vi "Run.vi"(8 "error in (no error)":errorcluster, 11 "Trigger in":refnum<class "Trigger.lvclass">) -> (0 "error out":errorcluster, 3 "Trigger out":refnum<class "Trigger.lvclass">)   [LabVIEW 2018, in "Trigger.lvclass"]
uses:
  Trigger.lvclass
  Trigger.lvclass/Trigger.ctl
  StateMachine/State Machine.lvclass
  Interface/Interface.lvclass
  Device/Device.lvclass
panel:
  out "resp":string
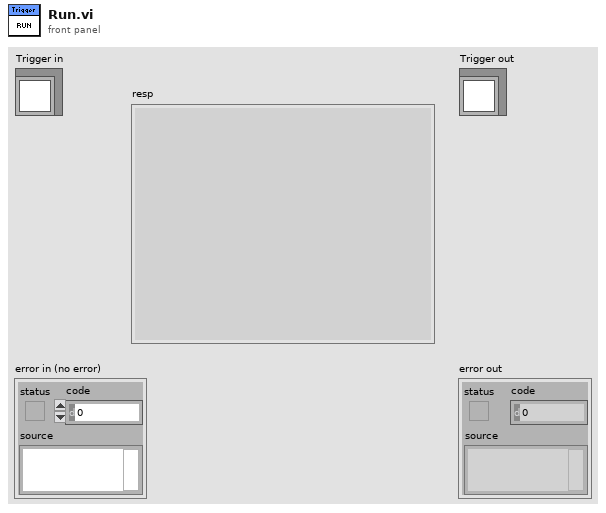
[diagram p1: front panel]
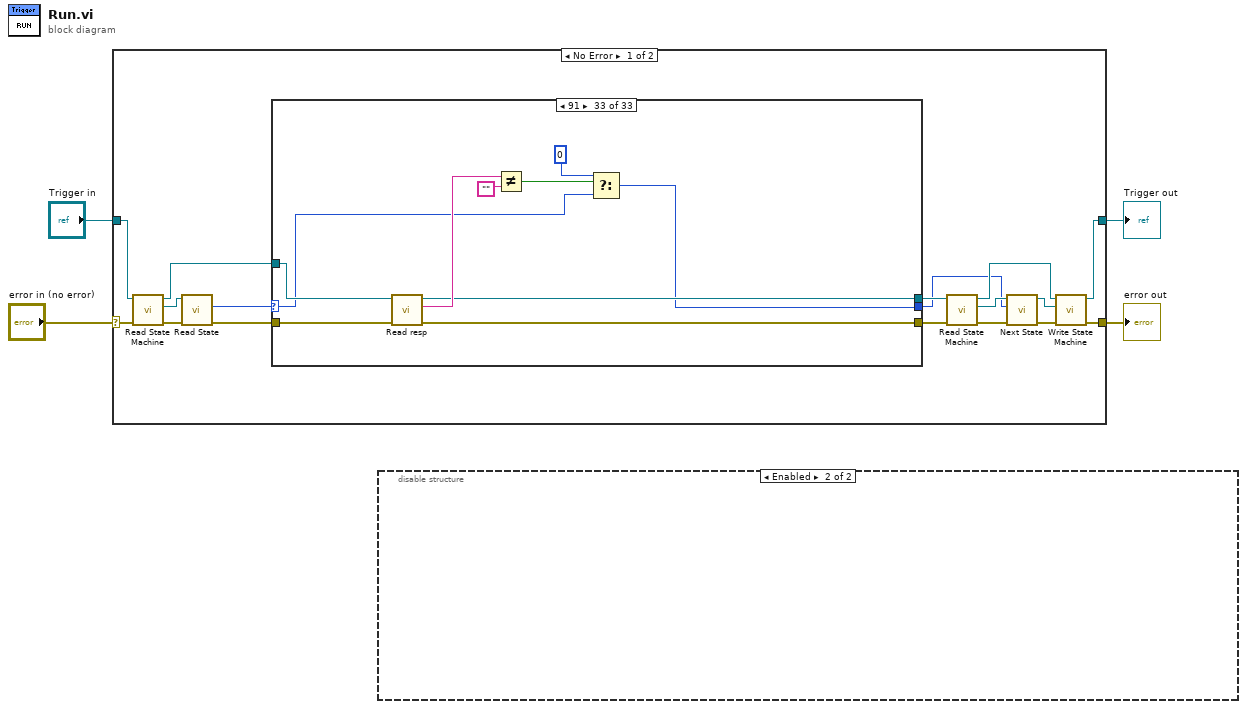
[diagram p0: block diagram]
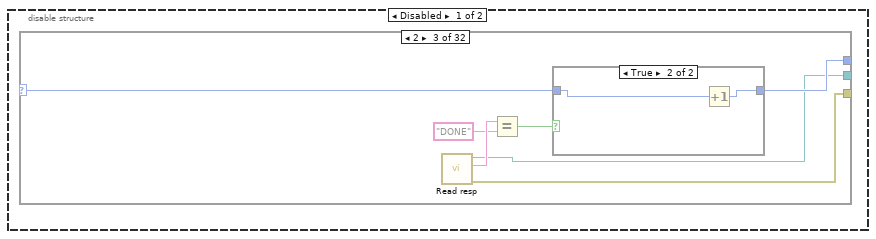
[diagram p2: hidden frame]
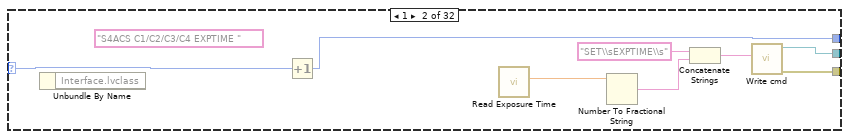
[diagram p4: hidden frame]
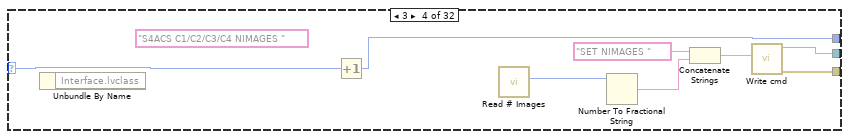
[diagram p6: hidden frame]
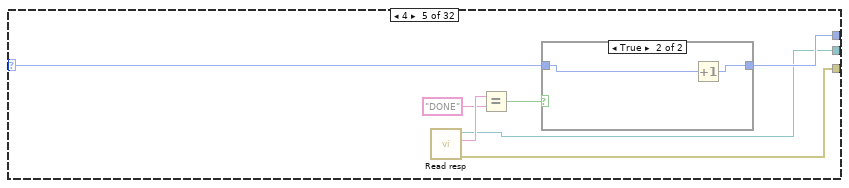
[diagram p7: hidden frame]
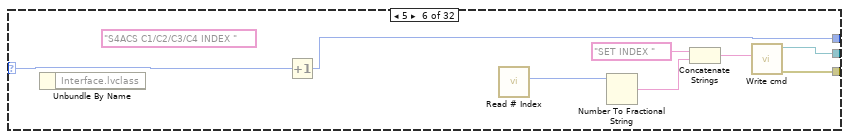
[diagram p9: hidden frame]
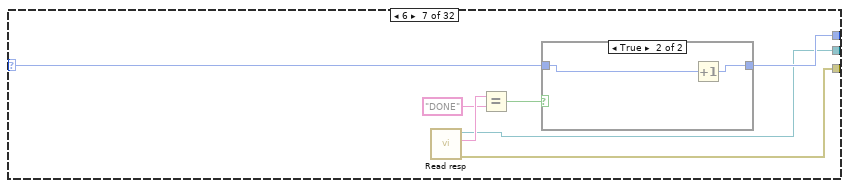
[diagram p10: hidden frame]
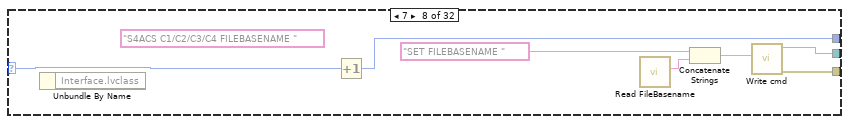
[diagram p12: hidden frame]
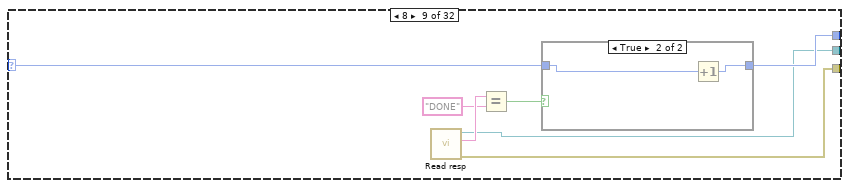
[diagram p13: hidden frame]
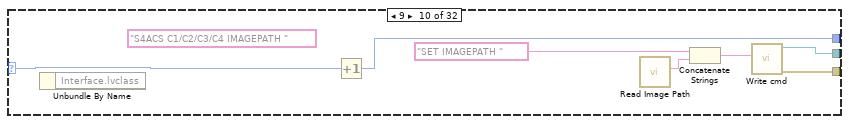
[diagram p15: hidden frame]
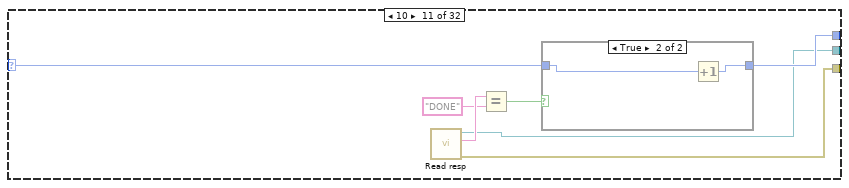
[diagram p16: hidden frame]
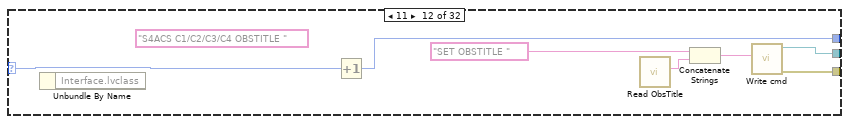
[diagram p18: hidden frame]
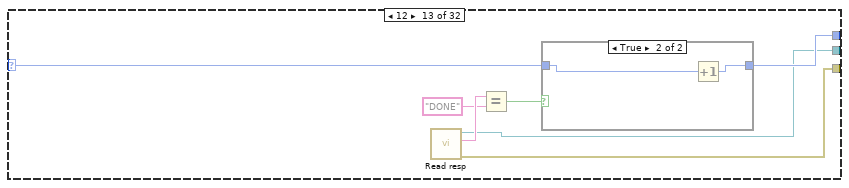
[diagram p19: hidden frame]
diagram:
  n1 = case shown="No Error" "error in (no error)" {
    selector: "error in (no error)" -> [w20 w479]
    tunnel: [w12 w479] -> w2
    tunnel: "Trigger in" -> [w21 w478]
    tunnel: [w11 w478] -> w1
    frame No Error {
      n2 = call-dynamic "Read State Machine.vi"("error in (no error)"=w20, "Device in"=w21) -> ("error out"=w18:errorcluster, "State Machine.lvclass"=w19:refnum<class "State Machine.lvclass">, "Device out"=w9:refnum<class "Trigger.lvclass">)  [unwired: 7 in]
      n3 = call-dynamic "Read State.vi"("error in (no error)"=w18, "State Machine in"=w19) -> ("error out"=w8:errorcluster, "State"=w10:i32)  [unwired: 7 in, 1 out]
      n4 = case shown="91" w10 {
        selector: w10 -> [_ w31 _ w48 w70 w82 w104 w116 w138 w150 w172 w184 w206 w218 w240 w252 w274 w286 w307 w323 w332 w340 _ w368 w381 w391 w404 w414 w427 w437 w451 w465 w469]
        tunnel: w9 -> [w23 w33 w44 w46 w78 w79 w112 w113 w146 w147 w180 w181 w214 w215 w248 w249 w282 w283 w314 w320 w329 w347 w362 w374 w389 w397 w412 w420 w435 w443 w458 w467 w477]
        tunnel: w8 -> [w22 w32 w43 w51 w77 w85 w111 w119 w145 w153 w179 w187 w213 w221 w247 w255 w281 w289 w313 w326 w335 w346 w366 w378 w388 w401 w411 w424 w434 w447 w457 w466 w476]
        tunnel: [w22 w25 w34 w50 w68 w84 w102 w118 w136 w152 w170 w186 w204 w220 w238 w254 w272 w288 w304 w325 w334 w345 w365 w377 w379 w400 w402 w423 w425 w446 w448 w459 w473] -> w7
        tunnel: [w23 w26 w35 w49 w69 w83 w103 w117 w137 w151 w171 w185 w205 w219 w239 w253 w273 w287 w305 w324 w333 w337 w364 w376 w380 w399 w403 w422 w426 w445 w449 w460 w472] -> w6
        tunnel: [0 ("State") w30 w39 w47 w75 w81 w109 w115 w143 w149 w177 w183 w211 w217 w245 w251 w279 w285 w311 w322 w331 w339 90 ("State") w367 w386 w390 w409 w413 w432 w436 w455 w464 w468] -> w5
        frame 0, Default {
        }
        frame 1 {
          n5 = Concatenate Strings("ST" ("cmd"), "\r") -> (w27:string)
          n6 = call-dynamic "Write cmd.vi"("error in (no error)"=w32, "cmd"=w27, "Device in"=w33) -> ("error out"=w25:errorcluster, "Device out"=w26:refnum<class "Trigger.lvclass">)  [unwired: 7 in]
          n7 = Increment(x=w31) -> (x+1=w30:i32)
        }
        frame 2 {
          n8 = call-dynamic "Read resp.vi"("error in (no error)"=w43, "Device in"=w44) -> ("error out"=w34:errorcluster, "resp"=w37:string, "Device out"=w38:refnum<class "Trigger.lvclass">)  [unwired: 7 in]
          "resp" <- w37
          n9 = Not Equal?(x=w37, y="") -> (x != y?=w42:bool)
          n10 = Bundle By Name(cluster=w38, "Trigger General Status"=w37) -> (w35:refnum<class "Trigger.lvclass">)
          n11 = Select(t=0, s=w42, f=2) -> (s? t:f=w39:i32)
        }
        frame 10 {
          n12 = Unbundle By Name(w46) -> ("enable A"=w45:bool)
          n13 = case shown="True" w45 {
            tunnel: w51 -> [w54 w67]
            tunnel: [w54 w66] -> w50
            tunnel: [w55 w65] -> w49
            tunnel: w48 -> [w56 w64]
            tunnel: [w53 w63] -> w47
            tunnel: w46 -> [w55 w60]
            frame False {
              n14 = Increment(x=w56) -> (x+1=w52:i32)
              n15 = Increment(x=w52) -> (x+1=w53:i32)
            }
            frame True {
              n16 = Unbundle By Name(w60) -> ("DelayA"=w59:string)
              n17 = Concatenate Strings("ADELAY " ("cmd"), w59, "m" ("cmd"), "\r") -> (w61:string)
              n18 = call-dynamic "Write cmd.vi"("error in (no error)"=w67, "cmd"=w61, "Device in"=w60) -> ("error out"=w66:errorcluster, "Device out"=w65:refnum<class "Trigger.lvclass">)  [unwired: 7 in]
              n19 = Increment(x=w64) -> (x+1=w63:i32)
            }
          }
        }
        frame 11 {
          w73 = "OK"
          n20 = call-dynamic "Read resp.vi"("error in (no error)"=w77, "Device in"=w78) -> ("error out"=w68:errorcluster, "resp"=w74:string, "Device out"=w69:refnum<class "Trigger.lvclass">)  [unwired: 7 in]
          n21 = Match Pattern(string=w74, regular expression=w73) -> (match substring=w72:string)  [unwired: 1 in, 3 out]
          n22 = Not Equal?(x=w72, y=w73) -> (x != y?=w76:bool)
          n23 = Increment(x=w70) -> (x+1=w71:i32)
          n24 = Select(t=w70, s=w76, f=w71) -> (s? t:f=w75:i32)
        }
        frame 12 {
          n25 = Unbundle By Name(w79) -> ("enable B"=w80:bool)
          n26 = case shown="True" w80 {
            tunnel: w85 -> [w89 w101]
            tunnel: [w89 w100] -> w84
            tunnel: [w90 w99] -> w83
            tunnel: w82 -> [w88 w98]
            tunnel: [w86 w97] -> w81
            tunnel: w79 -> [w90 w94]
            frame False {
              n27 = Increment(x=w88) -> (x+1=w87:i32)
              n28 = Increment(x=w87) -> (x+1=w86:i32)
            }
            frame True {
              n29 = Unbundle By Name(w94) -> ("DelayB"=w93:string)
              n30 = Concatenate Strings("BDELAY " ("cmd"), w93, "m" ("cmd"), "\r") -> (w95:string)
              n31 = call-dynamic "Write cmd.vi"("error in (no error)"=w101, "cmd"=w95, "Device in"=w94) -> ("error out"=w100:errorcluster, "Device out"=w99:refnum<class "Trigger.lvclass">)  [unwired: 7 in]
              n32 = Increment(x=w98) -> (x+1=w97:i32)
            }
          }
        }
        frame 13 {
          w107 = "OK"
          n33 = call-dynamic "Read resp.vi"("error in (no error)"=w111, "Device in"=w112) -> ("error out"=w102:errorcluster, "resp"=w108:string, "Device out"=w103:refnum<class "Trigger.lvclass">)  [unwired: 7 in]
          n34 = Match Pattern(string=w108, regular expression=w107) -> (match substring=w106:string)  [unwired: 1 in, 3 out]
          n35 = Not Equal?(x=w106, y=w107) -> (x != y?=w110:bool)
          n36 = Increment(x=w104) -> (x+1=w105:i32)
          n37 = Select(t=w104, s=w110, f=w105) -> (s? t:f=w109:i32)
        }
        frame 14 {
          n38 = Unbundle By Name(w113) -> ("enable C"=w114:bool)
          n39 = case shown="True" w114 {
            tunnel: w119 -> [w123 w135]
            tunnel: [w123 w134] -> w118
            tunnel: [w124 w133] -> w117
            tunnel: w116 -> [w122 w132]
            tunnel: [w121 w131] -> w115
            tunnel: w113 -> [w124 w128]
            frame False {
              n40 = Increment(x=w122) -> (x+1=w120:i32)
              n41 = Increment(x=w120) -> (x+1=w121:i32)
            }
            frame True {
              n42 = Unbundle By Name(w128) -> ("DelayC"=w127:string)
              n43 = Concatenate Strings("CDELAY " ("cmd"), w127, "m" ("cmd"), "\r") -> (w129:string)
              n44 = call-dynamic "Write cmd.vi"("error in (no error)"=w135, "cmd"=w129, "Device in"=w128) -> ("error out"=w134:errorcluster, "Device out"=w133:refnum<class "Trigger.lvclass">)  [unwired: 7 in]
              n45 = Increment(x=w132) -> (x+1=w131:i32)
            }
          }
        }
        frame 15 {
          w141 = "OK"
          n46 = call-dynamic "Read resp.vi"("error in (no error)"=w145, "Device in"=w146) -> ("error out"=w136:errorcluster, "resp"=w142:string, "Device out"=w137:refnum<class "Trigger.lvclass">)  [unwired: 7 in]
          n47 = Match Pattern(string=w142, regular expression=w141) -> (match substring=w140:string)  [unwired: 1 in, 3 out]
          n48 = Not Equal?(x=w140, y=w141) -> (x != y?=w144:bool)
          n49 = Increment(x=w138) -> (x+1=w139:i32)
          n50 = Select(t=w138, s=w144, f=w139) -> (s? t:f=w143:i32)
        }
        frame 16 {
          n51 = Unbundle By Name(w147) -> ("enable D"=w148:bool)
          n52 = case shown="False" w148 {
            tunnel: w153 -> [w157 w169]
            tunnel: [w157 w168] -> w152
            tunnel: [w158 w167] -> w151
            tunnel: w150 -> [w156 w166]
            tunnel: [w155 w165] -> w149
            tunnel: w147 -> [w158 w162]
            frame False {
              n53 = Increment(x=w156) -> (x+1=w154:i32)
              n54 = Increment(x=w154) -> (x+1=w155:i32)
            }
            frame True {
              n55 = Unbundle By Name(w162) -> ("DelayD"=w161:string)
              n56 = Concatenate Strings("DDELAY " ("cmd"), w161, "m" ("cmd"), "\r") -> (w163:string)
              n57 = call-dynamic "Write cmd.vi"("error in (no error)"=w169, "cmd"=w163, "Device in"=w162) -> ("error out"=w168:errorcluster, "Device out"=w167:refnum<class "Trigger.lvclass">)  [unwired: 7 in]
              n58 = Increment(x=w166) -> (x+1=w165:i32)
            }
          }
        }
        frame 17 {
          w175 = "OK"
          n59 = call-dynamic "Read resp.vi"("error in (no error)"=w179, "Device in"=w180) -> ("error out"=w170:errorcluster, "resp"=w176:string, "Device out"=w171:refnum<class "Trigger.lvclass">)  [unwired: 7 in]
          n60 = Match Pattern(string=w176, regular expression=w175) -> (match substring=w174:string)  [unwired: 1 in, 3 out]
          n61 = Not Equal?(x=w174, y=w175) -> (x != y?=w178:bool)
          n62 = Increment(x=w172) -> (x+1=w173:i32)
          n63 = Select(t=w172, s=w178, f=w173) -> (s? t:f=w177:i32)
        }
        frame 18 {
          n64 = Unbundle By Name(w181) -> ("enable A"=w182:bool)
          n65 = case shown="False" w182 {
            tunnel: w187 -> [w190 w203]
            tunnel: [w190 w202] -> w186
            tunnel: [w192 w201] -> w185
            tunnel: w184 -> [w191 w200]
            tunnel: [w188 w199] -> w183
            tunnel: w181 -> [w192 w196]
            frame False {
              n66 = Increment(x=w191) -> (x+1=w189:i32)
              n67 = Increment(x=w189) -> (x+1=w188:i32)
            }
            frame True {
              n68 = Unbundle By Name(w196) -> ("WidthA"=w195:string)
              n69 = Concatenate Strings("AWIDTH " ("cmd"), w195, "m" ("cmd"), "\r") -> (w197:string)
              n70 = call-dynamic "Write cmd.vi"("error in (no error)"=w203, "cmd"=w197, "Device in"=w196) -> ("error out"=w202:errorcluster, "Device out"=w201:refnum<class "Trigger.lvclass">)  [unwired: 7 in]
              n71 = Increment(x=w200) -> (x+1=w199:i32)
            }
          }
        }
        frame 19 {
          w209 = "OK"
          n72 = call-dynamic "Read resp.vi"("error in (no error)"=w213, "Device in"=w214) -> ("error out"=w204:errorcluster, "resp"=w210:string, "Device out"=w205:refnum<class "Trigger.lvclass">)  [unwired: 7 in]
          n73 = Match Pattern(string=w210, regular expression=w209) -> (match substring=w208:string)  [unwired: 1 in, 3 out]
          n74 = Not Equal?(x=w208, y=w209) -> (x != y?=w212:bool)
          n75 = Increment(x=w206) -> (x+1=w207:i32)
          n76 = Select(t=w206, s=w212, f=w207) -> (s? t:f=w211:i32)
        }
        frame 20 {
          n77 = Unbundle By Name(w215) -> ("enable B"=w216:bool)
          n78 = case shown="False" w216 {
            tunnel: w221 -> [w225 w237]
            tunnel: [w225 w236] -> w220
            tunnel: [w226 w235] -> w219
            tunnel: w218 -> [w224 w234]
            tunnel: [w223 w233] -> w217
            tunnel: w215 -> [w226 w230]
            frame False {
              n79 = Increment(x=w224) -> (x+1=w222:i32)
              n80 = Increment(x=w222) -> (x+1=w223:i32)
            }
            frame True {
              n81 = Unbundle By Name(w230) -> ("WidthB"=w229:string)
              n82 = Concatenate Strings("BWIDTH " ("cmd"), w229, "m" ("cmd"), "\r") -> (w231:string)
              n83 = call-dynamic "Write cmd.vi"("error in (no error)"=w237, "cmd"=w231, "Device in"=w230) -> ("error out"=w236:errorcluster, "Device out"=w235:refnum<class "Trigger.lvclass">)  [unwired: 7 in]
              n84 = Increment(x=w234) -> (x+1=w233:i32)
            }
          }
        }
        frame 21 {
          w243 = "OK"
          n85 = call-dynamic "Read resp.vi"("error in (no error)"=w247, "Device in"=w248) -> ("error out"=w238:errorcluster, "resp"=w244:string, "Device out"=w239:refnum<class "Trigger.lvclass">)  [unwired: 7 in]
          n86 = Match Pattern(string=w244, regular expression=w243) -> (match substring=w242:string)  [unwired: 1 in, 3 out]
          n87 = Not Equal?(x=w242, y=w243) -> (x != y?=w246:bool)
          n88 = Increment(x=w240) -> (x+1=w241:i32)
          n89 = Select(t=w240, s=w246, f=w241) -> (s? t:f=w245:i32)
        }
        frame 22 {
          n90 = Unbundle By Name(w249) -> ("enable C"=w250:bool)
          n91 = case shown="False" w250 {
            tunnel: w255 -> [w258 w271]
            tunnel: [w258 w270] -> w254
            tunnel: [w259 w269] -> w253
            tunnel: w252 -> [w260 w268]
            tunnel: [w257 w267] -> w251
            tunnel: w249 -> [w259 w264]
            frame False {
              n92 = Increment(x=w260) -> (x+1=w256:i32)
              n93 = Increment(x=w256) -> (x+1=w257:i32)
            }
            frame True {
              n94 = Unbundle By Name(w264) -> ("WidthC"=w263:string)
              n95 = Concatenate Strings("CWIDTH " ("cmd"), w263, "m" ("cmd"), "\r") -> (w265:string)
              n96 = call-dynamic "Write cmd.vi"("error in (no error)"=w271, "cmd"=w265, "Device in"=w264) -> ("error out"=w270:errorcluster, "Device out"=w269:refnum<class "Trigger.lvclass">)  [unwired: 7 in]
              n97 = Increment(x=w268) -> (x+1=w267:i32)
            }
          }
        }
        frame 23 {
          w277 = "OK"
          n98 = call-dynamic "Read resp.vi"("error in (no error)"=w281, "Device in"=w282) -> ("error out"=w272:errorcluster, "resp"=w278:string, "Device out"=w273:refnum<class "Trigger.lvclass">)  [unwired: 7 in]
          n99 = Match Pattern(string=w278, regular expression=w277) -> (match substring=w276:string)  [unwired: 1 in, 3 out]
          n100 = Not Equal?(x=w276, y=w277) -> (x != y?=w280:bool)
          n101 = Increment(x=w274) -> (x+1=w275:i32)
          n102 = Select(t=w274, s=w280, f=w275) -> (s? t:f=w279:i32)
        }
        frame 24 {
          n103 = Unbundle By Name(w283) -> ("enable D"=w284:bool)
          n104 = case shown="True" w284 {
            tunnel: w289 -> [w291 w303]
            tunnel: [w291 w302] -> w288
            tunnel: [w292 w301] -> w287
            tunnel: w286 -> [_ w300]
            tunnel: [90 w299] -> w285
            tunnel: w283 -> [w292 w296]
            frame False {
            }
            frame True {
              n105 = Unbundle By Name(w296) -> ("WidthD"=w295:string)
              n106 = Concatenate Strings("DWIDTH " ("cmd"), w295, "m" ("cmd"), "\r") -> (w297:string)
              n107 = call-dynamic "Write cmd.vi"("error in (no error)"=w303, "cmd"=w297, "Device in"=w296) -> ("error out"=w302:errorcluster, "Device out"=w301:refnum<class "Trigger.lvclass">)  [unwired: 7 in]
              n108 = Increment(x=w300) -> (x+1=w299:i32)
            }
          }
        }
        frame 25 {
          w309 = "OK"
          n109 = call-dynamic "Read resp.vi"("error in (no error)"=w313, "Device in"=w314) -> ("error out"=w304:errorcluster, "resp"=w310:string, "Device out"=w305:refnum<class "Trigger.lvclass">)  [unwired: 7 in]
          n110 = Match Pattern(string=w310, regular expression=w309) -> (match substring=w308:string)  [unwired: 1 in, 3 out]
          n111 = Not Equal?(x=w308, y=w309) -> (x != y?=w312:bool)
          n112 = Select(t=w307, s=w312, f=u8 90) -> (s? t:f=w311:i32)
        }
        frame 30 {
          n113 = Unbundle By Name(w320) -> ("Trigger Mode Target"=w317:bool)
          n114 = Select(t="TRigger POs" ("cmd"), s=w317, f="TRigger REmote" ("cmd")) -> (s? t:f=w316:string)
          n115 = Increment(x=w323) -> (x+1=w322:i32)
          n116 = Concatenate Strings(w316, "\r") -> (w321:string)
          n117 = call-dynamic "Write cmd.vi"("error in (no error)"=w326, "cmd"=w321, "Device in"=w320) -> ("error out"=w325:errorcluster, "Device out"=w324:refnum<class "Trigger.lvclass">)  [unwired: 7 in]
        }
        frame 31 {
          n118 = Concatenate Strings("TRigger" ("string"), "\r") -> (w330:string)
          n119 = call-dynamic "Write cmd.vi"("error in (no error)"=w335, "cmd"=w330, "Device in"=w329) -> ("error out"=w334:errorcluster, "Device out"=w333:refnum<class "Trigger.lvclass">)  [unwired: 7 in]
          n120 = Increment(x=w332) -> (x+1=w331:i32)
        }
        frame 32 {
          w343 = "Trig"
          n121 = call-dynamic "Read resp.vi"("error in (no error)"=w346, "Device in"=w347) -> ("error out"=w345:errorcluster, "resp"=w344:string, "Device out"=w338:refnum<class "Trigger.lvclass">)  [unwired: 7 in]
          n122 = Match Pattern(string=w344, regular expression=w343) -> (match substring=w342:string, after substring=w336:string)  [unwired: 1 in, 2 out]
          n123 = Not Equal?(x=w342, y=w343) -> (x != y?=w341:bool)
          n124 = case shown="False" w341 {
            tunnel: w340 -> [_ w358]
            tunnel: [90 ("State") w358] -> w339
            tunnel: [w348 w357] -> w337
            tunnel: w338 -> [w356 w357]
            tunnel: w336 -> [w354 _]
            frame False {
              n125 = call <vilib>:"Trim Whitespace.vi"("string"=w354) -> ("trimmed string"=w352:string)  [unwired: 1 in]
              n126 = call <vilib>:"Space Constant.vi"() -> ("String"=w355:string)
              n127 = Match Pattern(string=w352, regular expression=w355) -> (before substring=w353:string, after substring=w350:string)  [unwired: 1 in, 2 out]
              n128 = Bundle By Name(cluster=w356, "Trigger Mode Status"=w353) -> (w351:refnum<class "Trigger.lvclass">)
              n129 = Bundle By Name(cluster=w351, "String output"=w350) -> (w348:refnum<class "Trigger.lvclass">)
            }
            frame True {
            }
          }
        }
        frame 40 {
          n130 = Concatenate Strings("FIre" ("string"), "\r") -> (w363:string)
          n131 = call-dynamic "Write cmd.vi"("error in (no error)"=w366, "cmd"=w363, "Device in"=w362) -> ("error out"=w365:errorcluster, "Device out"=w364:refnum<class "Trigger.lvclass">)  [unwired: 7 in]
        }
        frame 50 {
          n132 = Unbundle By Name(w374) -> ("enable A"=w372:bool)
          n133 = Select(t="aset on" ("string"), s=w372, f="aset off" ("string")) -> (s? t:f=w369:string)
          n134 = Concatenate Strings(w369, "\r") -> (w375:string)
          n135 = call-dynamic "Write cmd.vi"("error in (no error)"=w378, "cmd"=w375, "Device in"=w374) -> ("error out"=w377:errorcluster, "Device out"=w376:refnum<class "Trigger.lvclass">)  [unwired: 7 in]
          n136 = Increment(x=w368) -> (x+1=w367:i32)
        }
        frame 51 {
          w384 = "OK"
          n137 = call-dynamic "Read resp.vi"("error in (no error)"=w388, "Device in"=w389) -> ("error out"=w379:errorcluster, "resp"=w385:string, "Device out"=w380:refnum<class "Trigger.lvclass">)  [unwired: 7 in]
          n138 = Match Pattern(string=w385, regular expression=w384) -> (match substring=w383:string)  [unwired: 1 in, 3 out]
          n139 = Not Equal?(x=w383, y=w384) -> (x != y?=w387:bool)
          n140 = Increment(x=w381) -> (x+1=w382:i32)
          n141 = Select(t=w381, s=w387, f=w382) -> (s? t:f=w386:i32)
        }
        frame 52 {
          n142 = Unbundle By Name(w397) -> ("enable B"=w395:bool)
          n143 = Select(t="bset on" ("string"), s=w395, f="bset off" ("string")) -> (s? t:f=w392:string)
          n144 = Concatenate Strings(w392, "\r") -> (w398:string)
          n145 = call-dynamic "Write cmd.vi"("error in (no error)"=w401, "cmd"=w398, "Device in"=w397) -> ("error out"=w400:errorcluster, "Device out"=w399:refnum<class "Trigger.lvclass">)  [unwired: 7 in]
          n146 = Increment(x=w391) -> (x+1=w390:i32)
        }
        frame 53 {
          w407 = "OK"
          n147 = call-dynamic "Read resp.vi"("error in (no error)"=w411, "Device in"=w412) -> ("error out"=w402:errorcluster, "resp"=w408:string, "Device out"=w403:refnum<class "Trigger.lvclass">)  [unwired: 7 in]
          n148 = Match Pattern(string=w408, regular expression=w407) -> (match substring=w406:string)  [unwired: 1 in, 3 out]
          n149 = Not Equal?(x=w406, y=w407) -> (x != y?=w410:bool)
          n150 = Increment(x=w404) -> (x+1=w405:i32)
          n151 = Select(t=w404, s=w410, f=w405) -> (s? t:f=w409:i32)
        }
        frame 54 {
          n152 = Unbundle By Name(w420) -> ("enable C"=w418:bool)
          n153 = Select(t="cset on" ("string"), s=w418, f="cset off" ("string")) -> (s? t:f=w415:string)
          n154 = Concatenate Strings(w415, "\r") -> (w421:string)
          n155 = call-dynamic "Write cmd.vi"("error in (no error)"=w424, "cmd"=w421, "Device in"=w420) -> ("error out"=w423:errorcluster, "Device out"=w422:refnum<class "Trigger.lvclass">)  [unwired: 7 in]
          n156 = Increment(x=w414) -> (x+1=w413:i32)
        }
        frame 55 {
          w430 = "OK"
          n157 = call-dynamic "Read resp.vi"("error in (no error)"=w434, "Device in"=w435) -> ("error out"=w425:errorcluster, "resp"=w431:string, "Device out"=w426:refnum<class "Trigger.lvclass">)  [unwired: 7 in]
          n158 = Match Pattern(string=w431, regular expression=w430) -> (match substring=w429:string)  [unwired: 1 in, 3 out]
          n159 = Not Equal?(x=w429, y=w430) -> (x != y?=w433:bool)
          n160 = Increment(x=w427) -> (x+1=w428:i32)
          n161 = Select(t=w427, s=w433, f=w428) -> (s? t:f=w432:i32)
        }
        frame 56 {
          n162 = Unbundle By Name(w443) -> ("enable D"=w441:bool)
          n163 = Select(t="dset on" ("string"), s=w441, f="dset off" ("string")) -> (s? t:f=w438:string)
          n164 = Concatenate Strings(w438, "\r") -> (w444:string)
          n165 = call-dynamic "Write cmd.vi"("error in (no error)"=w447, "cmd"=w444, "Device in"=w443) -> ("error out"=w446:errorcluster, "Device out"=w445:refnum<class "Trigger.lvclass">)  [unwired: 7 in]
          n166 = Increment(x=w437) -> (x+1=w436:i32)
        }
        frame 57 {
          w453 = "OK"
          n167 = call-dynamic "Read resp.vi"("error in (no error)"=w457, "Device in"=w458) -> ("error out"=w448:errorcluster, "resp"=w454:string, "Device out"=w449:refnum<class "Trigger.lvclass">)  [unwired: 7 in]
          n168 = Match Pattern(string=w454, regular expression=w453) -> (match substring=w452:string)  [unwired: 1 in, 3 out]
          n169 = Not Equal?(x=w452, y=w453) -> (x != y?=w456:bool)
          n170 = Select(t=w451, s=w456, f=90) -> (s? t:f=w455:i32)
        }
        frame 90 {
          # "Aplica todos os comandos pendentes."
          n171 = Concatenate Strings("IN" ("cmd"), "\r") -> (w461:string)
          n172 = call-dynamic "Write cmd.vi"("error in (no error)"=w466, "cmd"=w461, "Device in"=w467) -> ("error out"=w459:errorcluster, "Device out"=w460:refnum<class "Trigger.lvclass">)  [unwired: 7 in]
          n173 = Increment(x=w465) -> (x+1=w464:i32)
        }
        frame 91 {
          n174 = call-dynamic "Read resp.vi"("error in (no error)"=w476, "Device in"=w477) -> ("error out"=w473:errorcluster, "resp"=w475:string, "Device out"=w472:refnum<class "Trigger.lvclass">)  [unwired: 7 in]
          n175 = Not Equal?(x=w475, y="") -> (x != y?=w470:bool)
          n176 = Select(t=0, s=w470, f=w469) -> (s? t:f=w468:i32)
        }
      }
      n177 = call-dynamic "Read State Machine.vi"("error in (no error)"=w7, "Device in"=w6) -> ("error out"=w14:errorcluster, "State Machine.lvclass"=w16:refnum<class "State Machine.lvclass">, "Device out"=w15:refnum<class "Trigger.lvclass">)  [unwired: 7 in]
      n178 = call "Next State.vi"("error in (no error)"=w14, "New_State"=w5, "State Machine in"=w16) -> ("error out"=w13:errorcluster, "State Machine out"=w17:refnum<class "State Machine.lvclass">)  [unwired: 7 in]
      n179 = call-dynamic "Write State Machine.vi"("error in (no error)"=w13, "State Machine.lvclass"=w17, "Device in"=w15) -> ("error out"=w12:errorcluster, "Device out"=w11:refnum<class "Trigger.lvclass">)  [unwired: 7 in]
    }
    frame Error {
    }
  }
  "error out" <- w2
  "Trigger out" <- w1
  n180 = disable-structure shown="Enabled" {
    frame Disabled {
      n181 = case shown="2" {
        selector: _ -> [w480 w482 w489 w500 w507 w518 w525 w537 w542 w554 w559 w571 w576 w588 w593 w605 w610 w620 w624 w635 w642 w648 w657 w672 w687 w702 w717 w732 w747 w762 w776 _]
        tunnel: [_ w487 w490 w505 w508 w523 w526 w540 w543 w557 w560 w574 w577 w591 w594 w608 w611 w622 w625 w637 w643 w650 w658 _ _ _ _ _ _ _ _ _] -> _
        tunnel: [_ w488 w491 w506 w509 w524 w527 w541 w544 w558 w561 w575 w578 w592 w595 w609 w612 w623 w626 w638 w641 w651 w654 w669 w684 w699 w714 w729 w744 w759 _ _] -> _
        tunnel: [w480 w483 w492 w501 w510 w519 w528 w538 w545 w555 w562 w572 w579 w589 w596 w606 w613 w621 w627 w636 w644 w649 w659 w667 w682 w697 w712 w727 w742 w757 w772 u8 0 ("State")] -> _
        frame 0, Default {
        }
        frame 1 {
          (unwired) "S4ACS C1/C2/C3/C4 EXPTIME " ("cmd")
          n182 = Unbundle By Name() -> ()  [unwired: 1 in, 1 out]
          n183 = Increment(x=w482) -> (x+1=w483:u8)
          n184 = call "Read Exposure Time.vi"() -> ("Exposure Time"=w486:dbl)  [unwired: 9 in, 2 out]
          n185 = Number To Fractional String(number=w486) -> (F-format string=w485:string)  [unwired: 3 in]
          n186 = Concatenate Strings("SET\\sEXPTIME\\s" ("cmd"), w485) -> (w484:string)
          n187 = call-dynamic "Write cmd.vi"("cmd"=w484) -> ("error out"=w487:errorcluster, "Device out"=w488:refnum<class "Device.lvclass">)  [unwired: 9 in]
        }
        frame 2 {
          n188 = call-dynamic "Read resp.vi"() -> ("error out"=w490:errorcluster, "resp"=w495:string, "Device out"=w491:refnum<class "Device.lvclass">)  [unwired: 9 in]
          n189 = Equal?(x=w495, y="DONE") -> (x = y?=w493:bool)
          n190 = case shown="True" w493 {
            tunnel: [w496 w497] -> w492
            tunnel: w489 -> [w496 w498]
            frame False {
            }
            frame True {
              n191 = Increment(x=w498) -> (x+1=w497:u8)
            }
          }
        }
        frame 3 {
          (unwired) "S4ACS C1/C2/C3/C4 NIMAGES " ("cmd")
          n192 = Unbundle By Name() -> ()  [unwired: 1 in, 1 out]
          n193 = Increment(x=w500) -> (x+1=w501:u8)
          n194 = call-dynamic "Read # Images.vi"() -> ("# Images"=w504:u32)  [unwired: 9 in, 2 out]
          n195 = Number To Fractional String(number=w504) -> (F-format string=w503:string)  [unwired: 3 in]
          n196 = Concatenate Strings("SET NIMAGES " ("cmd"), w503) -> (w502:string)
          n197 = call-dynamic "Write cmd.vi"("cmd"=w502) -> ("error out"=w505:errorcluster, "Device out"=w506:refnum<class "Device.lvclass">)  [unwired: 9 in]
        }
        frame 4 {
          n198 = call-dynamic "Read resp.vi"() -> ("error out"=w508:errorcluster, "resp"=w513:string, "Device out"=w509:refnum<class "Device.lvclass">)  [unwired: 9 in]
          n199 = Equal?(x=w513, y="DONE") -> (x = y?=w511:bool)
          n200 = case shown="True" w511 {
            tunnel: [w514 w515] -> w510
            tunnel: w507 -> [w514 w516]
            frame False {
            }
            frame True {
              n201 = Increment(x=w516) -> (x+1=w515:u8)
            }
          }
        }
        frame 5 {
          (unwired) "S4ACS C1/C2/C3/C4 INDEX " ("cmd")
          n202 = Unbundle By Name() -> ()  [unwired: 1 in, 1 out]
          n203 = Increment(x=w518) -> (x+1=w519:u8)
          n204 = call-dynamic "Read # Index.vi"() -> ("# Index"=w522:u32)  [unwired: 9 in, 2 out]
          n205 = Number To Fractional String(number=w522) -> (F-format string=w521:string)  [unwired: 3 in]
          n206 = Concatenate Strings("SET INDEX " ("cmd"), w521) -> (w520:string)
          n207 = call-dynamic "Write cmd.vi"("cmd"=w520) -> ("error out"=w523:errorcluster, "Device out"=w524:refnum<class "Device.lvclass">)  [unwired: 9 in]
        }
        frame 6 {
          n208 = call-dynamic "Read resp.vi"() -> ("error out"=w526:errorcluster, "resp"=w531:string, "Device out"=w527:refnum<class "Device.lvclass">)  [unwired: 9 in]
          n209 = Equal?(x=w531, y="DONE") -> (x = y?=w529:bool)
          n210 = case shown="True" w529 {
            tunnel: [w532 w533] -> w528
            tunnel: w525 -> [w532 w534]
            frame False {
            }
            frame True {
              n211 = Increment(x=w534) -> (x+1=w533:u8)
            }
          }
        }
        frame 7 {
          (unwired) "S4ACS C1/C2/C3/C4 FILEBASENAME " ("cmd")
          n212 = Unbundle By Name() -> ()  [unwired: 1 in, 1 out]
          n213 = Increment(x=w537) -> (x+1=w538:u8)
          n214 = call-dynamic "Read FileBasename.vi"() -> ("FileBasename"=w535:string)  [unwired: 9 in, 2 out]
          n215 = Concatenate Strings("SET FILEBASENAME " ("cmd"), w535) -> (w539:string)
          n216 = call-dynamic "Write cmd.vi"("cmd"=w539) -> ("error out"=w540:errorcluster, "Device out"=w541:refnum<class "Device.lvclass">)  [unwired: 9 in]
        }
        frame 8 {
          n217 = call-dynamic "Read resp.vi"() -> ("error out"=w543:errorcluster, "resp"=w548:string, "Device out"=w544:refnum<class "Device.lvclass">)  [unwired: 9 in]
          n218 = Equal?(x=w548, y="DONE") -> (x = y?=w546:bool)
          n219 = case shown="True" w546 {
            tunnel: [w549 w550] -> w545
            tunnel: w542 -> [w549 w551]
            frame False {
            }
            frame True {
              n220 = Increment(x=w551) -> (x+1=w550:u8)
            }
          }
        }
        frame 9 {
          (unwired) "S4ACS C1/C2/C3/C4 IMAGEPATH " ("cmd")
          n221 = Unbundle By Name() -> ()  [unwired: 1 in, 1 out]
          n222 = Increment(x=w554) -> (x+1=w555:u8)
          n223 = call-dynamic "Read Image Path.vi"() -> ("Image Path"=w552:string)  [unwired: 9 in, 2 out]
          n224 = Concatenate Strings("SET IMAGEPATH " ("cmd"), w552) -> (w556:string)
          n225 = call-dynamic "Write cmd.vi"("cmd"=w556) -> ("error out"=w557:errorcluster, "Device out"=w558:refnum<class "Device.lvclass">)  [unwired: 9 in]
        }
        frame 10 {
          n226 = call-dynamic "Read resp.vi"() -> ("error out"=w560:errorcluster, "resp"=w565:string, "Device out"=w561:refnum<class "Device.lvclass">)  [unwired: 9 in]
          n227 = Equal?(x=w565, y="DONE") -> (x = y?=w563:bool)
          n228 = case shown="True" w563 {
            tunnel: [w566 w567] -> w562
            tunnel: w559 -> [w566 w568]
            frame False {
            }
            frame True {
              n229 = Increment(x=w568) -> (x+1=w567:u8)
            }
          }
        }
        frame 11 {
          (unwired) "S4ACS C1/C2/C3/C4 OBSTITLE " ("cmd")
          n230 = Unbundle By Name() -> ()  [unwired: 1 in, 1 out]
          n231 = Increment(x=w571) -> (x+1=w572:u8)
          n232 = call-dynamic "Read ObsTitle.vi"() -> ("ObsTitle"=w569:string)  [unwired: 9 in, 2 out]
          n233 = Concatenate Strings("SET OBSTITLE " ("cmd"), w569) -> (w573:string)
          n234 = call-dynamic "Write cmd.vi"("cmd"=w573) -> ("error out"=w574:errorcluster, "Device out"=w575:refnum<class "Device.lvclass">)  [unwired: 9 in]
        }
        frame 12 {
          n235 = call-dynamic "Read resp.vi"() -> ("error out"=w577:errorcluster, "resp"=w582:string, "Device out"=w578:refnum<class "Device.lvclass">)  [unwired: 9 in]
          n236 = Equal?(x=w582, y="DONE") -> (x = y?=w580:bool)
          n237 = case shown="True" w580 {
            tunnel: [w583 w584] -> w579
            tunnel: w576 -> [w583 w585]
            frame False {
            }
            frame True {
              n238 = Increment(x=w585) -> (x+1=w584:u8)
            }
          }
        }
        frame 13 {
          (unwired) "S4ACS C1/C2/C3/C4 COMMENTS " ("cmd")
          n239 = Unbundle By Name() -> ()  [unwired: 1 in, 1 out]
          n240 = Increment(x=w588) -> (x+1=w589:u8)
          n241 = call-dynamic "Read Comments.vi"() -> ("Comments"=w586:string)  [unwired: 9 in, 2 out]
          n242 = Concatenate Strings("SET COMMENTS " ("cmd"), w586) -> (w590:string)
          n243 = call-dynamic "Write cmd.vi"("cmd"=w590) -> ("error out"=w591:errorcluster, "Device out"=w592:refnum<class "Device.lvclass">)  [unwired: 9 in]
        }
        frame 14 {
          n244 = call-dynamic "Read resp.vi"() -> ("error out"=w594:errorcluster, "resp"=w599:string, "Device out"=w595:refnum<class "Device.lvclass">)  [unwired: 9 in]
          n245 = Equal?(x=w599, y="DONE") -> (x = y?=w597:bool)
          n246 = case shown="True" w597 {
            tunnel: [w600 w601] -> w596
            tunnel: w593 -> [w600 w602]
            frame False {
            }
            frame True {
              n247 = Increment(x=w602) -> (x+1=w601:u8)
            }
          }
        }
        frame 15 {
          (unwired) "S4ACS C1/C2/C3/C4 DS9 " ("cmd")
          n248 = Unbundle By Name() -> ()  [unwired: 1 in, 1 out]
          n249 = Increment(x=w605) -> (x+1=w606:u8)
          n250 = call-dynamic "Read DS9.vi"() -> ("DS9"=w603:string)  [unwired: 9 in, 2 out]
          n251 = Concatenate Strings("SET DS9 " ("cmd"), w603) -> (w607:string)
          n252 = call-dynamic "Write cmd.vi"("cmd"=w607) -> ("error out"=w608:errorcluster, "Device out"=w609:refnum<class "Device.lvclass">)  [unwired: 9 in]
        }
        frame 16 {
          n253 = call-dynamic "Read resp.vi"() -> ("error out"=w611:errorcluster, "resp"=w616:string, "Device out"=w612:refnum<class "Device.lvclass">)  [unwired: 9 in]
          n254 = Equal?(x=w616, y="DONE") -> (x = y?=w614:bool)
          n255 = case shown="True" w614 {
            tunnel: [w617 u8 50 ("State")] -> w613
            tunnel: w610 -> [w617 _]
            frame False {
            }
            frame True {
            }
          }
        }
        frame 50 {
          (unwired) "S4ACS C1/C2/C3/C4 EXPOSE " ("cmd")
          n256 = Increment(x=w620) -> (x+1=w621:u8)
          n257 = call-dynamic "Write cmd.vi"("cmd"="EXPOSE ") -> ("error out"=w622:errorcluster, "Device out"=w623:refnum<class "Device.lvclass">)  [unwired: 9 in]
        }
        frame 51 {
          n258 = call-dynamic "Read resp.vi"() -> ("error out"=w625:errorcluster, "resp"=w630:string, "Device out"=w626:refnum<class "Device.lvclass">)  [unwired: 9 in]
          n259 = Equal?(x=w630, y="DONE") -> (x = y?=w628:bool)
          n260 = case shown="True" w628 {
            tunnel: [w631 w632] -> w627
            tunnel: w624 -> [w631 w633]
            frame False {
            }
            frame True {
              n261 = Increment(x=w633) -> (x+1=w632:u8)
            }
          }
        }
        frame 52 {
          (unwired) "S4ACS C1/C2/C3/C4 STATUS " ("cmd")
          n262 = Increment(x=w635) -> (x+1=w636:u8)
          n263 = call-dynamic "Write cmd.vi"("cmd"="STATUS ") -> ("error out"=w637:errorcluster, "Device out"=w638:refnum<class "Device.lvclass">)  [unwired: 9 in]
        }
        frame 53 {
          # "Extrair todos os parametros da respsota de STATUS e\natualizar a informação na classe Channel."
          n264 = case shown="True" FALSE {
            tunnel: [w645 u8 0 ("State")] -> w644
            tunnel: w642 -> [w645 _]
            frame False {
            }
            frame True {
            }
          }
          n265 = call-dynamic "Read resp.vi"() -> ("error out"=w643:errorcluster)  [unwired: 9 in, 2 out]
          n266 = Bundle By Name("Texp"=0.0 ("Status.Texp")) -> (w641:cluster{})  [unwired: 1 in]
        }
        frame 100 {
          (unwired) "S4ACS C1/C2/C3/C4 NIMAGES " ("cmd")
          n267 = Increment(x=w648) -> (x+1=w649:u8)
          n268 = call-dynamic "Write cmd.vi"("cmd"="STATUS") -> ("error out"=w650:errorcluster, "Device out"=w651:refnum<class "Device.lvclass">)  [unwired: 9 in]
        }
        frame 101 {
          w653 = "\r\n"
          n269 = call-dynamic "Read resp.vi"() -> ("error out"=w658:errorcluster, "resp"=w652:string, "Device out"=w655:refnum<class "Device.lvclass">)  [unwired: 9 in]
          n270 = Match Pattern(string=w652, regular expression=w653) -> (match substring=w656:string)  [unwired: 1 in, 3 out]
          n271 = Equal?(x=w656, y=w653) -> (x = y?=w660:bool)
          n272 = case shown="True" w660 {
            tunnel: [u8 0 w663] -> w659
            tunnel: w657 -> [_ w664]
            tunnel: w655 -> [w662 _]
            tunnel: [w662 w666] -> w654
            tunnel: w652 -> [_ w665]
            frame False {
            }
            frame True {
              n273 = Bundle By Name("lastStatus"=w665) -> (w666:cluster{})  [unwired: 1 in]
              n274 = Increment(x=w664) -> (x+1=w663:u8)
            }
          }
        }
        frame 102 {
          w671 = "EXPTIME "
          n275 = Unbundle By Name() -> ()  [unwired: 1 in, 1 out]
          n276 = Match Pattern(regular expression=w671) -> (match substring=w670:string, after substring=w668:string)  [unwired: 2 in, 2 out]
          n277 = Equal?(x=w670, y=w671) -> (x = y?=w674:bool)
          n278 = case shown="True" w674 {
            tunnel: [w675 w676] -> w673
            tunnel: w672 -> [w675 w676]
            tunnel: [_ w680] -> w669
            tunnel: w668 -> [_ w678]
            frame False {
            }
            frame True {
              n279 = call <vilib>:"Space Constant.vi"() -> ("String"=w679:string)
              n280 = Match Pattern(string=w678, regular expression=w679) -> (before substring=w677:string)  [unwired: 1 in, 3 out]
              n281 = Fract/Exp String To Number(string=w677) -> (number=w681:dbl)  [unwired: 3 in, 1 out]
              n282 = Bundle By Name("Texp"=w681) -> (w680:cluster{})  [unwired: 1 in]
            }
          }
          n283 = Increment(x=w673) -> (x+1=w667:u8)
        }
        frame 103 {
          w686 = "NIMAGES "
          n284 = Unbundle By Name() -> ()  [unwired: 1 in, 1 out]
          n285 = Match Pattern(regular expression=w686) -> (match substring=w685:string, after substring=w683:string)  [unwired: 2 in, 2 out]
          n286 = Equal?(x=w685, y=w686) -> (x = y?=w689:bool)
          n287 = case shown="True" w689 {
            tunnel: [w690 w691] -> w688
            tunnel: w687 -> [w690 w691]
            tunnel: [_ w695] -> w684
            tunnel: w683 -> [_ w693]
            frame False {
            }
            frame True {
              n288 = call <vilib>:"Space Constant.vi"() -> ("String"=w694:string)
              n289 = Match Pattern(string=w693, regular expression=w694) -> (before substring=w692:string)  [unwired: 1 in, 3 out]
              n290 = Fract/Exp String To Number(string=w692) -> (number=w696:dbl)  [unwired: 3 in, 1 out]
              n291 = Bundle By Name("Nimages"=w696) -> (w695:cluster{})  [unwired: 1 in]
            }
          }
          n292 = Increment(x=w688) -> (x+1=w682:u8)
        }
        frame 104 {
          w701 = "INITIAL_LINE "
          n293 = Unbundle By Name() -> ()  [unwired: 1 in, 1 out]
          n294 = Match Pattern(regular expression=w701) -> (match substring=w700:string, after substring=w698:string)  [unwired: 2 in, 2 out]
          n295 = Equal?(x=w700, y=w701) -> (x = y?=w704:bool)
          n296 = case shown="True" w704 {
            tunnel: [w705 w706] -> w703
            tunnel: w702 -> [w705 w706]
            tunnel: [_ w710] -> w699
            tunnel: w698 -> [_ w708]
            frame False {
            }
            frame True {
              n297 = call <vilib>:"Space Constant.vi"() -> ("String"=w709:string)
              n298 = Match Pattern(string=w708, regular expression=w709) -> (before substring=w707:string)  [unwired: 1 in, 3 out]
              n299 = Fract/Exp String To Number(string=w707) -> (number=w711:dbl)  [unwired: 3 in, 1 out]
              n300 = Bundle By Name("InitialLine"=w711) -> (w710:cluster{})  [unwired: 1 in]
            }
          }
          n301 = Increment(x=w703) -> (x+1=w697:u8)
        }
        frame 105 {
          w716 = "FINAL_LINE "
          n302 = Unbundle By Name() -> ()  [unwired: 1 in, 1 out]
          n303 = Match Pattern(regular expression=w716) -> (match substring=w715:string, after substring=w713:string)  [unwired: 2 in, 2 out]
          n304 = Equal?(x=w715, y=w716) -> (x = y?=w719:bool)
          n305 = case shown="True" w719 {
            tunnel: [w720 w721] -> w718
            tunnel: w717 -> [w720 w721]
            tunnel: [_ w725] -> w714
            tunnel: w713 -> [_ w723]
            frame False {
            }
            frame True {
              n306 = call <vilib>:"Space Constant.vi"() -> ("String"=w724:string)
              n307 = Match Pattern(string=w723, regular expression=w724) -> (before substring=w722:string)  [unwired: 1 in, 3 out]
              n308 = Fract/Exp String To Number(string=w722) -> (number=w726:dbl)  [unwired: 3 in, 1 out]
              n309 = Bundle By Name("FinalLine"=w726) -> (w725:cluster{})  [unwired: 1 in]
            }
          }
          n310 = Increment(x=w718) -> (x+1=w712:u8)
        }
        frame 106 {
          w731 = "INITIAL_COLUMN "
          n311 = Unbundle By Name() -> ()  [unwired: 1 in, 1 out]
          n312 = Match Pattern(regular expression=w731) -> (match substring=w730:string, after substring=w728:string)  [unwired: 2 in, 2 out]
          n313 = Equal?(x=w730, y=w731) -> (x = y?=w734:bool)
          n314 = case shown="False" w734 {
            tunnel: [w735 w736] -> w733
            tunnel: w732 -> [w735 w736]
            tunnel: [_ w740] -> w729
            tunnel: w728 -> [_ w738]
            frame False {
            }
            frame True {
              n315 = call <vilib>:"Space Constant.vi"() -> ("String"=w739:string)
              n316 = Match Pattern(string=w738, regular expression=w739) -> (before substring=w737:string)  [unwired: 1 in, 3 out]
              n317 = Fract/Exp String To Number(string=w737) -> (number=w741:dbl)  [unwired: 3 in, 1 out]
              n318 = Bundle By Name("InitialColumn"=w741) -> (w740:cluster{})  [unwired: 1 in]
            }
          }
          n319 = Increment(x=w733) -> (x+1=w727:u8)
        }
        frame 107 {
          w746 = "FINAL_COLUMN "
          n320 = Unbundle By Name() -> ()  [unwired: 1 in, 1 out]
          n321 = Match Pattern(regular expression=w746) -> (match substring=w745:string, after substring=w743:string)  [unwired: 2 in, 2 out]
          n322 = Equal?(x=w745, y=w746) -> (x = y?=w749:bool)
          n323 = case shown="True" w749 {
            tunnel: [w750 w751] -> w748
            tunnel: w747 -> [w750 w751]
            tunnel: [_ w755] -> w744
            tunnel: w743 -> [_ w753]
            frame False {
            }
            frame True {
              n324 = call <vilib>:"Space Constant.vi"() -> ("String"=w754:string)
              n325 = Match Pattern(string=w753, regular expression=w754) -> (before substring=w752:string)  [unwired: 1 in, 3 out]
              n326 = Fract/Exp String To Number(string=w752) -> (number=w756:dbl)  [unwired: 3 in, 1 out]
              n327 = Bundle By Name("FinalColumn"=w756) -> (w755:cluster{})  [unwired: 1 in]
            }
          }
          n328 = Increment(x=w748) -> (x+1=w742:u8)
        }
        frame 108 {
          w761 = "EM_GAIN "
          n329 = Unbundle By Name() -> ()  [unwired: 1 in, 1 out]
          n330 = Match Pattern(regular expression=w761) -> (match substring=w760:string, after substring=w758:string)  [unwired: 2 in, 2 out]
          n331 = Equal?(x=w760, y=w761) -> (x = y?=w764:bool)
          n332 = case shown="True" w764 {
            tunnel: [w765 w766] -> w763
            tunnel: w762 -> [w765 w766]
            tunnel: [_ w770] -> w759
            tunnel: w758 -> [_ w768]
            frame False {
            }
            frame True {
              n333 = call <vilib>:"Space Constant.vi"() -> ("String"=w769:string)
              n334 = Match Pattern(string=w768, regular expression=w769) -> (before substring=w767:string)  [unwired: 1 in, 3 out]
              n335 = Fract/Exp String To Number(string=w767) -> (number=w771:dbl)  [unwired: 3 in, 1 out]
              n336 = Bundle By Name("EmGain"=w771) -> (w770:cluster{})  [unwired: 1 in]
            }
          }
          n337 = Increment(x=w763) -> (x+1=w757:u8)
        }
        frame 109 {
          w775 = "COOLER "
          n338 = Match Pattern(regular expression=w775) -> (match substring=w774:string, after substring=w773:string)  [unwired: 2 in, 2 out]
          n339 = Equal?(x=w774, y=w775) -> (x = y?=w778:bool)
          n340 = case shown="False" w778 {
            tunnel: [w779 w780] -> w777
            tunnel: w776 -> [w779 w780]
            tunnel: w773 -> [_ w783]
            frame False {
            }
            frame True {
              n341 = call <vilib>:"Space Constant.vi"() -> ("String"=w784:string)
              n342 = Match Pattern(string=w783, regular expression=w784) -> (before substring=w782:string)  [unwired: 1 in, 3 out]
              n343 = Equal?(x=w782, y="ON") -> ()  [unwired: 1 out]
            }
          }
          n344 = Increment(x=w777) -> (x+1=w772:u8)
        }
        frame 110 {
        }
      }
    }
    frame Enabled {
    }
  }
